vi "写校验.vi"(11 "数据输入":u8[](array[numeric])) -> (3 "data输出":u8[](array[numeric]))   [LabVIEW 2012]
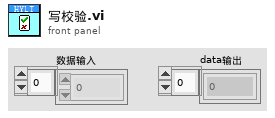
[diagram p1: front panel]
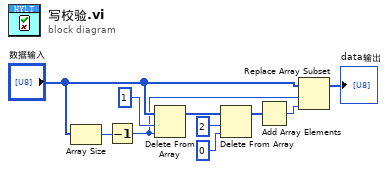
[diagram p0: block diagram]
diagram:
  n1 = Array Size(array="数据输入") -> (size(s)=w7:i32)
  n2 = Decrement(x=w7) -> (x-1=w2:i32)
  n3 = Delete From Array(array="数据输入", length=1 ("长度"), index=w2) -> (array with subset deleted=w9:u8[])  [unwired: 1 out]
  n4 = Delete From Array(array=w9, length=2 ("长度"), index=0 ("索引")) -> (array with subset deleted=w8:u8[])  [unwired: 1 out]
  n5 = Add Array Elements(numeric array=w8) -> (sum=w3:u8)
  n6 = Replace Array Subset(array="数据输入", new element=w3, index=w2) -> (→"data输出":u8[])
